vi "VecBuilder_3x1Fill.vi"(9 "R2":dbl, 10 "R1":dbl, 11 "R0":dbl) -> (3 "output matrix":T1)   [LabVIEW 2019, in "Trajectory_Library.lvlib"]
doc: "Creates a new LINEAR SYSTEM data cluster with the specified values. \n\n\nInputs: \n - XXX -- XXX.\n\nOutputs:\n - XXX -- XXX."
uses:
  Trajectory_Library.lvlib
  <vilib>/Analysis/Matrix/Datatypes/RealMatrix.ctl
  <vilib>/Analysis/Matrix/NI_Matrix.lvlib
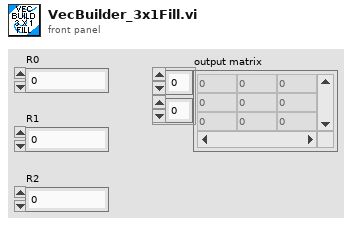
[diagram p1: front panel]
types:
  T1 = typedef "NI_Matrix.lvlib/RealMatrix.ctl" = dbl[][]
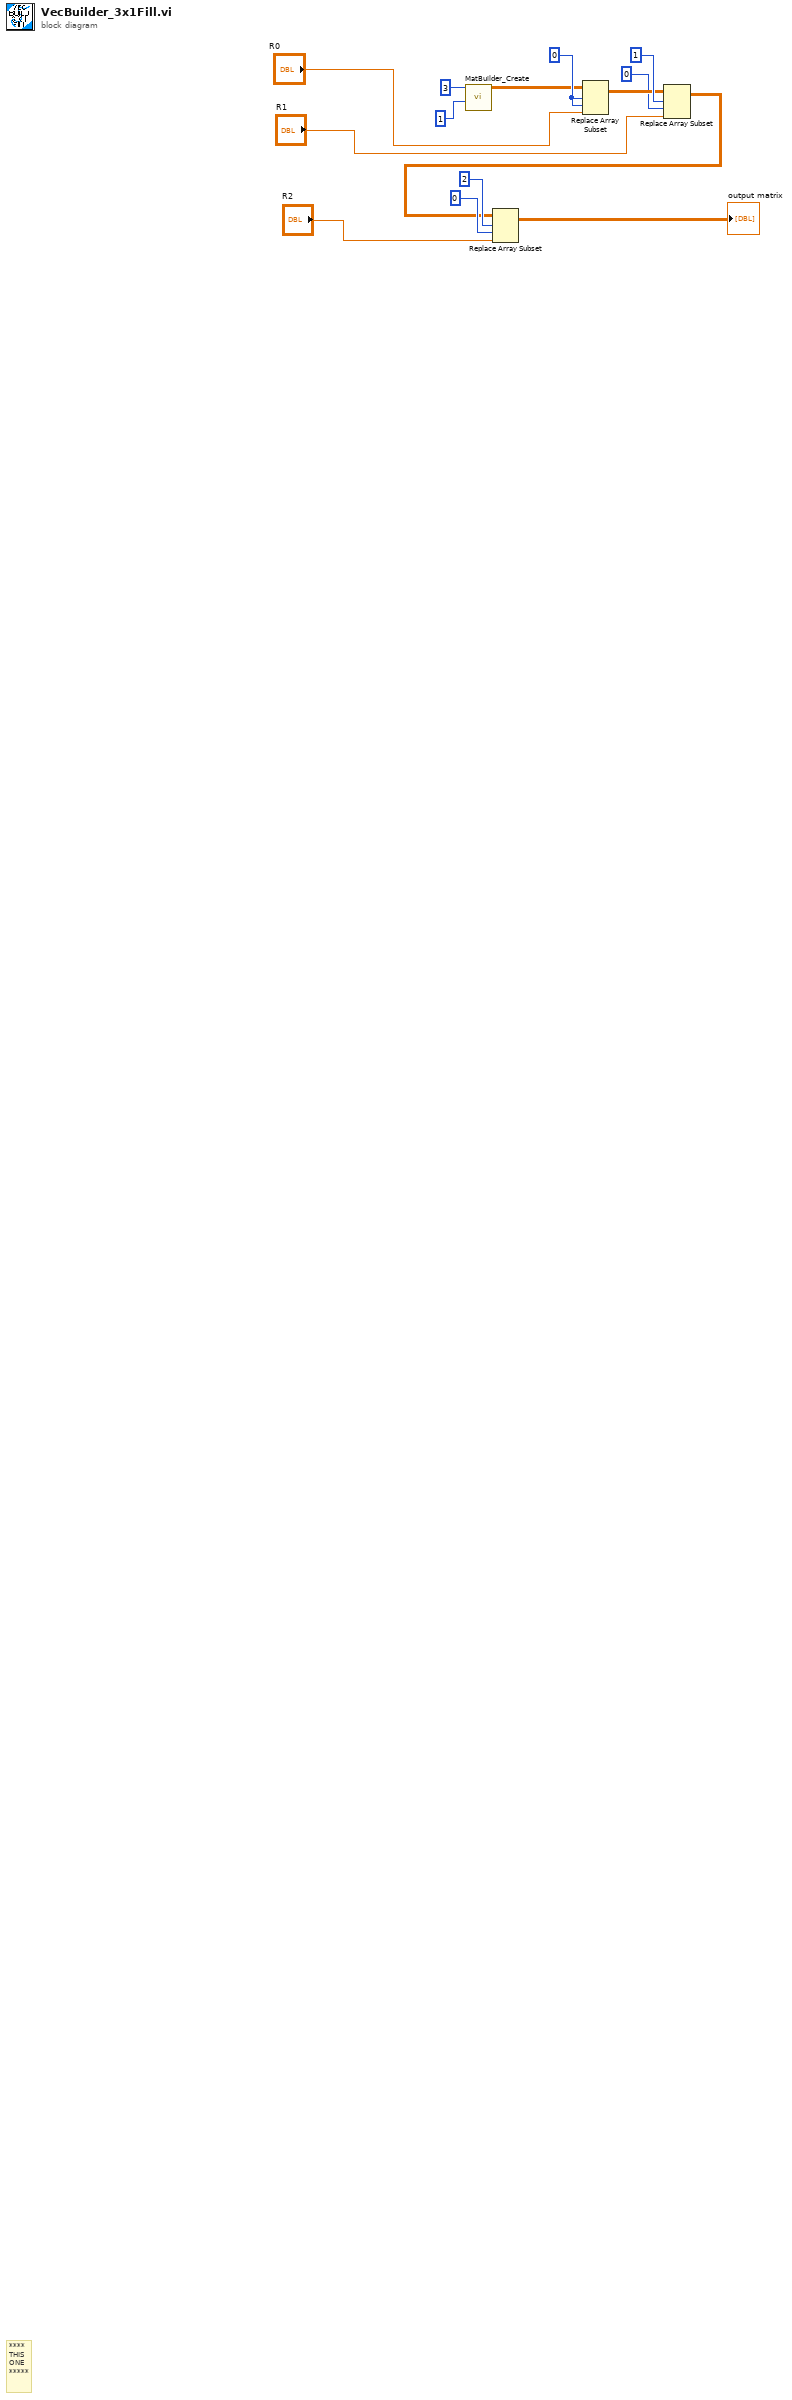
[diagram p0: block diagram]
diagram:
  w14 = 0 ("index (col)")
  # "****\nTHIS\nONE\n*****"
  n1 = call "MatBuilder_Create.vi"("Columns"=1, "Rows"=3) -> ("output matrix"=w1:T1)  [unwired: 9 in]
  n2 = Replace Array Subset(array=w1, new element="R0", index (row)=w14, index (col)=w14) -> (w12:T1)
  n3 = Replace Array Subset(array=w12, new element="R1", index (row)=1 ("index (col)"), index (col)=0 ("disabled index (col)")) -> (w5:T1)
  n4 = Replace Array Subset(array=w5, new element="R2", index (row)=2 ("index (col)"), index (col)=0 ("disabled index (col)")) -> (→"output matrix":T1)
